vi "sample_PowerMeter.vi"() -> ()   [LabVIEW 2012]
panel:
  out "Power":dbl
  out "New Data":bool
  out "Watts":dbl
  out "Sensor SN":string
  out "Sensor Name":string
  in  "stop":bool
  out "Readout value":dbl(slide) scale=9e-07..0.0001
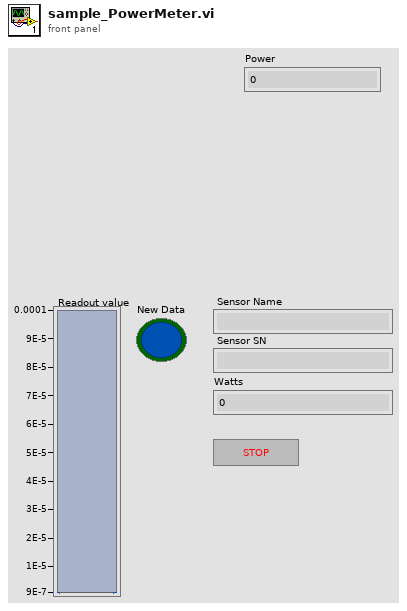
[diagram p1: front panel]
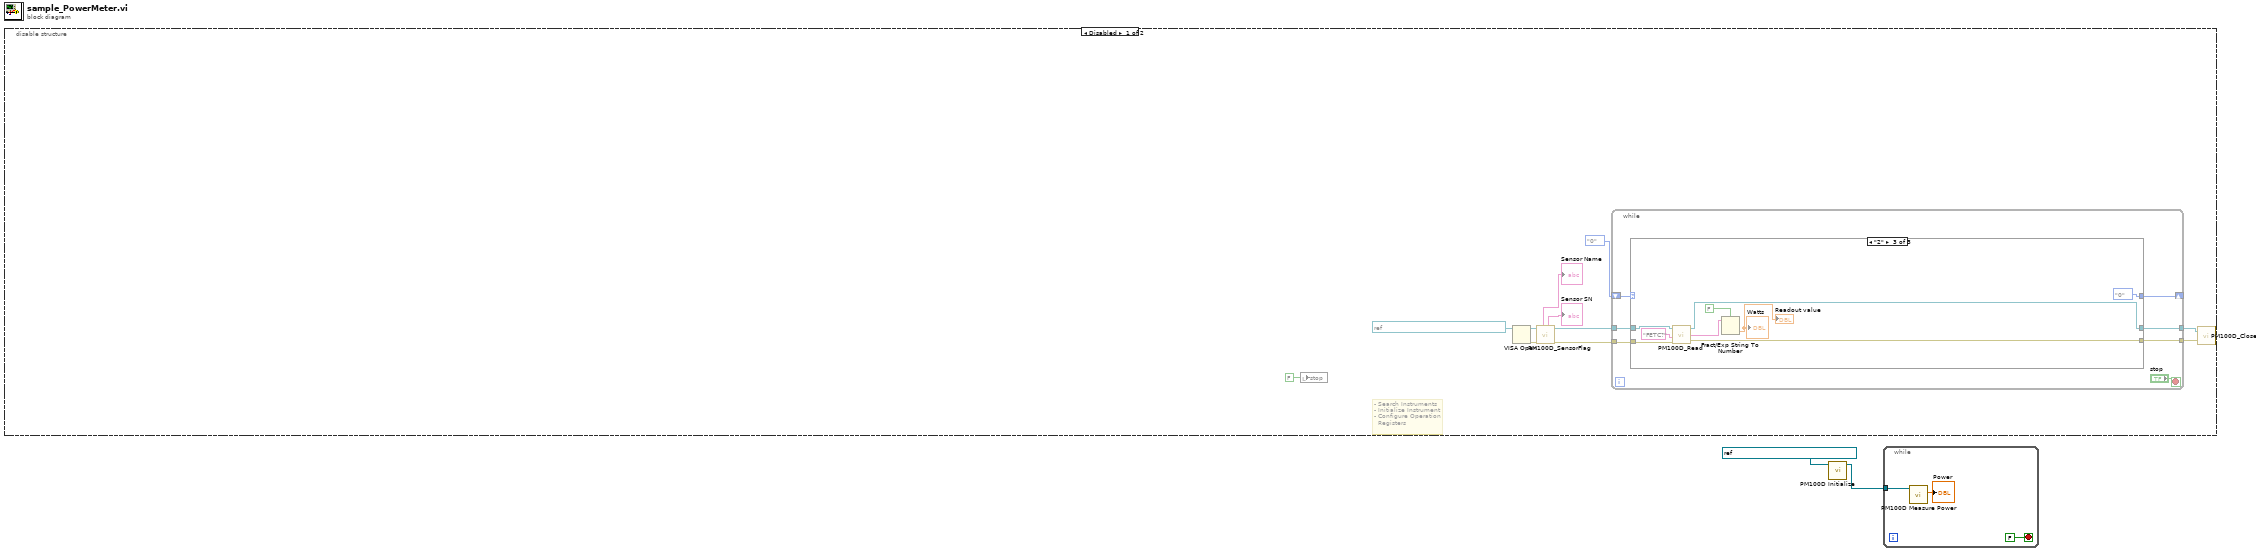
[diagram p0: block diagram]
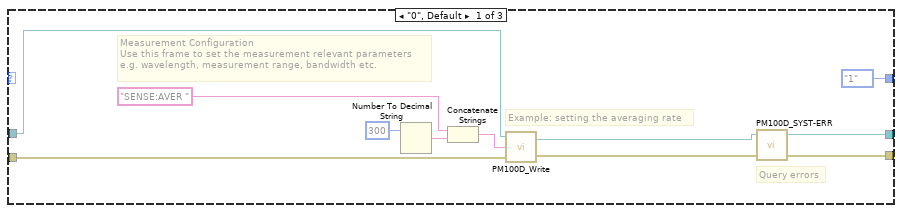
[diagram p2: hidden frame]
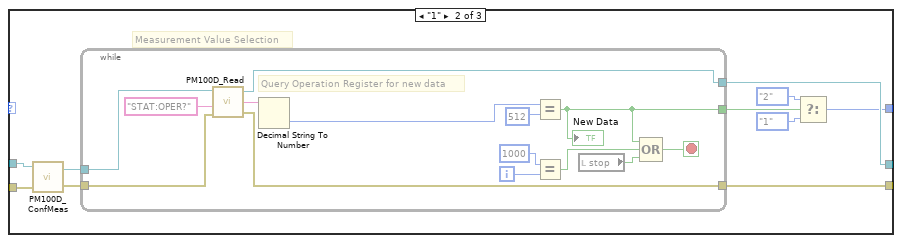
[diagram p3: hidden frame]
diagram:
  n1 = disable-structure shown="Disabled" {
    frame Disabled {
      # "- Search Instruments\n- Initialize Instrument\n- Configure Operation\n  Registers"
      n2 = local write "stop"(FALSE ("stop")) -> ()
      n3 = VISA Open(VISA resource name=refnum<visa-resource-name> "USB0::0x1313::0x8078::P0006758::INSTR") -> (VISA resource name=w6:refnum<visa-resource-name>, error out=w5:errorcluster)  [unwired: 4 in]
      n4 = call "PM100D_SensorFlag.vi"("error in (no error)"=w5, "VISA in"=w6) -> ("error out"=w12:errorcluster, "VISA out"=w13:refnum<visa-resource-name>, "sn"=→"Sensor SN":string, "name"=→"Sensor Name":string)  [unwired: 2 in, 4 out]
      n5 = while {
        tunnel: w13 -> [w20]
        tunnel: w12 -> [w19]
        shift-right: [w16] -> _
        shift-left: enum16{"0", "1", "2"}."0" -> [w17]
        tunnel: [w15] -> w10
        tunnel: [w14] -> w9
        stop <- "stop" stop-if-true
        n6 = case shown="\"2\"" w17 {
          tunnel: w20 -> [w28 w41 w62]
          tunnel: w19 -> [w24 w40 w61]
          tunnel: [enum16{"0", "1", "2"}."1" w35 enum16{"0", "1", "2"}."0"] -> w16
          tunnel: [w22 w37 w60] -> w15
          tunnel: [w21 w36 w56] -> w14
          frame "0", Default {
            # "Query errors"
            # "Example: setting the averaging rate"
            # "Measurement Configuration\nUse this frame to set the measurement relevant parameters\ne.g. wavelength, measurement range, bandwidth etc."
            n7 = Number To Decimal String(number=300 ("Averaging Rate")) -> (decimal integer string=w30:string)  [unwired: 1 in]
            n8 = Concatenate Strings("SENSE:AVER " ("string"), w30) -> (w27:string)
            n9 = call "PM100D_Write.vi"("error in (no error)"=w24, "Command"=w27, "VISA in"=w28) -> ("error out"=w25:errorcluster, "VISA out"=w26:refnum<visa-resource-name>)
            n10 = call "PM100D_SYST-ERR.vi"("error out 2"=w25, "VISA In"=w26) -> ("error out"=w21:errorcluster, "VISA Out"=w22:refnum<visa-resource-name>)  [unwired: 1 in, 1 out]
          }
          frame "1" {
            # "Measurement Value Selection"
            n11 = call "PM100D_ConfMeas.vi"("error in"=w40, "VISA In"=w41) -> ("error out"=w38:errorcluster, "dup VISA session"=w39:refnum<visa-resource-name>)  [unwired: 1 in]
            n12 = while {
              tunnel: w39 -> [w51]
              tunnel: w38 -> [w50]
              tunnel: [w49] -> w37
              tunnel: [w48] -> w36
              tunnel: [w42] -> w32
              i -> [w44]
              stop <- w46 stop-if-true
              # "Query Operation Register for new data"
              n13 = call "PM100D_Read.vi"("error in (no error)"=w50, "Command"="STAT:OPER?", "VISA in"=w51) -> ("error out"=w48:errorcluster, "ReadValue"=w54:string, "VISA out"=w49:refnum<visa-resource-name>)  [unwired: 1 in]
              n14 = Decimal String To Number(string=w54) -> (number=w53:i32)  [unwired: 2 in, 1 out]
              n15 = Equal?(x=w53, y=512) -> (x = y?=w42:bool)
              "New Data" <- w42
              n16 = Equal?(x=1000 ("Timeout [ms]"), y=w44) -> (x = y?=w43:bool)
              n17 = local read "stop"() -> (w47:bool)
              n18 = Compound Arithmetic op=OR(w42, w43, w47) -> (w46:bool)
            }
            n19 = Select(t=enum16{"0", "1", "2"}."2", s=w32, f=enum16{"0", "1", "2"}."1") -> (s? t:f=w35:enum16{"0", "1", "2"})
          }
          frame "2" {
            n20 = call "PM100D_Read.vi"("error in (no error)"=w61, "Command"="FETC?", "VISA in"=w62) -> ("error out"=w56:errorcluster, "ReadValue"=w59:string, "VISA out"=w60:refnum<visa-resource-name>)  [unwired: 1 in]
            n21 = Fract/Exp String To Number(use system decimal point (T)=FALSE, string=w59) -> (number=→"Readout value" →"Watts":dbl)  [unwired: 2 in, 1 out]
          }
        }
      }
      n22 = call "PM100D_Close.vi"("error in (no error)"=w9, "VISA resource name"=w10) -> ()  [unwired: 2 in]
    }
    frame Enabled {
    }
  }
  n23 = call <instrlib>:"PM100D Initialize.vi"("resource name"=refnum<visa-resource-name> "USB0::0x1313::0x8078::P0006758::INSTR") -> ("instrument handle out"=w1:refnum<visa-resource-name>)  [unwired: 9 in, 1 out]
  n24 = while {
    tunnel: w1 -> [w66]
    stop <- FALSE stop-if-true
    n25 = call <instrlib>:"PM100D Measure Power.vi"("instrument handle"=w66) -> ("Power"=→"Power":dbl)  [unwired: 8 in, 2 out]
  }
